vi "invertarray.vi"(11 "number":dbl[](array[numeric])) -> (3 "output":dbl[](array[numeric]))   [LabVIEW 2020]
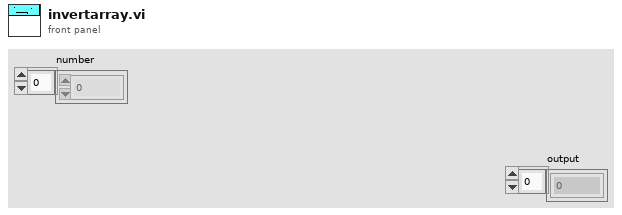
[diagram p1: front panel]
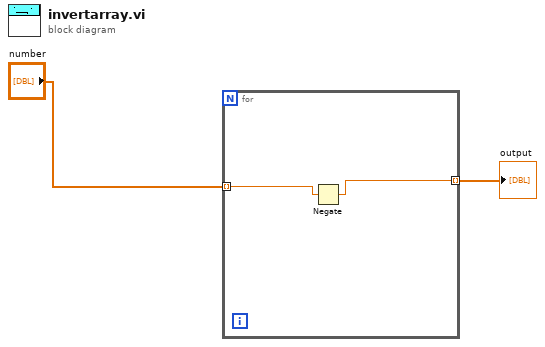
[diagram p0: block diagram]
diagram:
  n1 = for {
    tunnel: "number" -> [w4] mode=indexing
    tunnel: [w3] -> w1 mode=indexing
    n2 = Negate(x=w4) -> (-x=w3:dbl)
  }
  "output" <- w1
